vi "File Save Waveform.vi"(8 "error in (no error)":errorcluster, 10 "Waveforms":waveform(dbl)[](array[waveform]), 11 "File Path":path) -> (0 "error out":errorcluster)   [LabVIEW 2017]
doc: "This VI converts then saves the waveform into a CSV.\n\nI didn't use the default method that LabVIEW use to save waveform. I changed it in such a way that the waveform can be displayed on Scatter XY format when opened in excel."
uses:
  <vilib>/Utility/file.llb/Write Delimited Spreadsheet (string).vi
  <vilib>/Utility/file.llb/Write Delimited Spreadsheet (DBL).vi
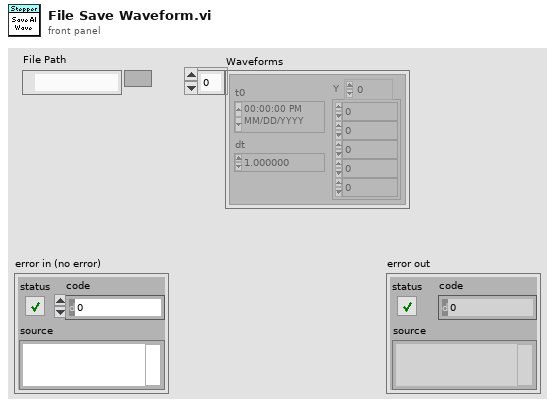
[diagram p1: front panel]
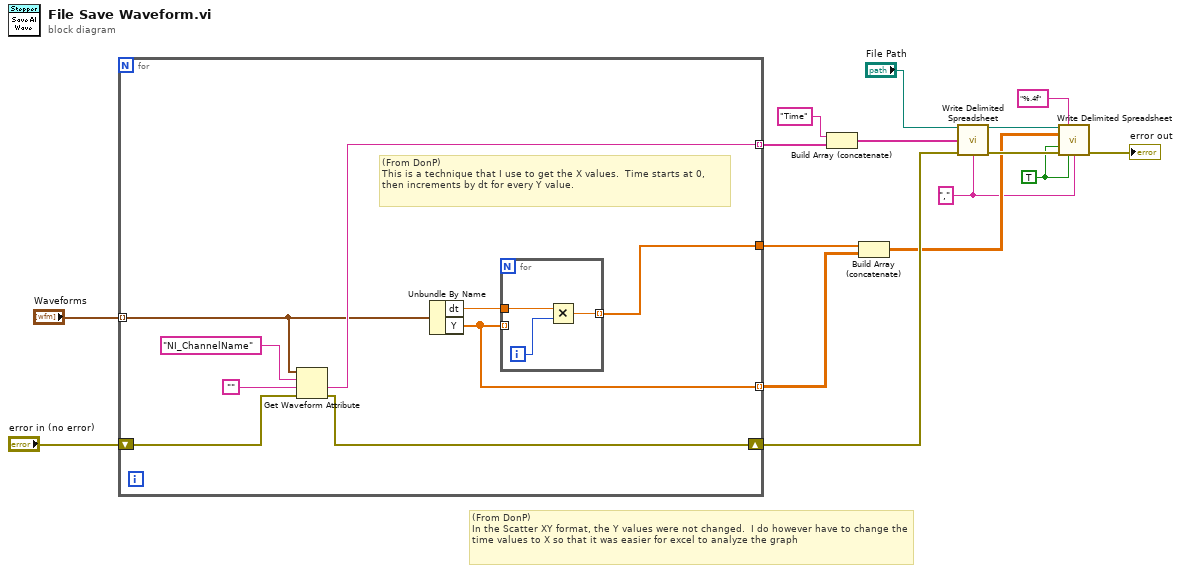
[diagram p0: block diagram]
diagram:
  w7 = TRUE ("append to file? (new file:F)")
  w6 = "," ("delimiter (\\t)")
  # "(From DonP)\nIn the Scatter XY format, the Y values were not changed.  I do however have to change the time values to X so that it was easier for excel to analyze the graph"
  n1 = for {
    tunnel: "Waveforms" -> [w21] mode=indexing
    shift-right: [w17] -> w11
    shift-left: "error in (no error)" -> [w23]
    tunnel: [w22] -> w3 mode=indexing
    tunnel: [w19] -> w14
    tunnel: [w18] -> w13 mode=indexing
    # "(From DonP)\nThis is a technique that I use to get the X values.  Time starts at 0, then increments by dt for every Y value."
    n2 = Get Waveform Attribute(4:w23, 5:"", 6:"NI_ChannelName" ("name"), 7:w21) -> (0:w17:errorcluster, 1:w22:string)  [unwired: 2 out]
    n3 = Unbundle By Name(w21) -> ("dt"=w20:dbl, "Y"=w18:dbl[])
    n4 = for {
      tunnel: w18 -> [_] mode=indexing
      tunnel: w20 -> [w28]
      tunnel: [w26] -> w19 mode=indexing
      i -> [w27]
      n5 = Multiply(x=w28, y=w27) -> (x*y=w26:dbl)
    }
  }
  n6 = Build Array (concatenate)("Time", w3) -> (w2:string[])
  n7 = Build Array (concatenate)(w14, w13) -> (w8:dbl[][])
  n8 = call-poly <vilib>:"Write Delimited Spreadsheet.vi"("file path (dialog if empty)"="File Path", "1D data"=w2, "error in (no error)"=w11, "delimiter (\\t)"=w6) -> ("new file path (Not A Path if cancelled)"=w10:path, "error out"=w9:errorcluster)  [unwired: 10 in]
  n9 = call-poly <vilib>:"Write Delimited Spreadsheet.vi"("file path (dialog if empty)"=w10, "format (%.3f)"="%.4f", "2D data"=w8, "append to file? (new file:F)"=w7, "error in (no error)"=w9, "transpose? (no:F)"=w7, "delimiter (\\t)"=w6) -> ("error out"=→"error out":errorcluster)  [unwired: 7 in, 1 out]
